vi "DOE Zero DC Clamp Meter.vi"(11 "Uncorrected Voltage":dbl) -> (3 "Corrected Voltage":dbl)   [LabVIEW 2019]
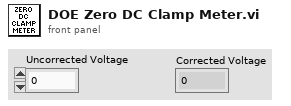
[diagram p1: front panel]
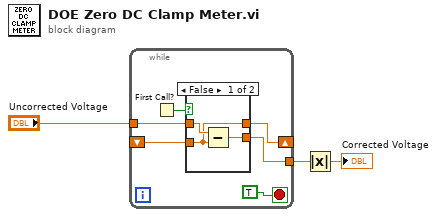
[diagram p0: block diagram]
diagram:
  n1 = while {
    shift-right: [w6] -> _
    shift-left: _ -> [w5]
    tunnel: "Uncorrected Voltage" -> [w8]
    tunnel: [w4] -> w2
    stop <- TRUE stop-if-true
    n2 = First Call?() -> (First Call?: T/F=w7:bool)
    n3 = case shown="False" w7 {
      tunnel: w8 -> [w12 w13]
      tunnel: [w11 w13] -> w6
      tunnel: w5 -> [w11 _]
      tunnel: [w10 w13] -> w4
      frame False {
        n4 = Subtract(x=w12, y=w11) -> (x-y=w10:dbl)
      }
      frame True {
      }
    }
  }
  n5 = Absolute Value(x=w2) -> (abs(x)=→"Corrected Voltage":dbl)
